vi "Get Type Code (Variant).vi"(6 "error in (no error)":errorcluster, 9 "value":variant) -> (0 "error out":errorcluster, 2 "type code":T1=enum."Bool", 3 "value dup":variant)   [LabVIEW 2020, in "Value.lvlib"]
uses:
  Value.lvlib
  Type Code.ctl
  <vilib>/Utility/Data Type/NI_Data Type.lvlib
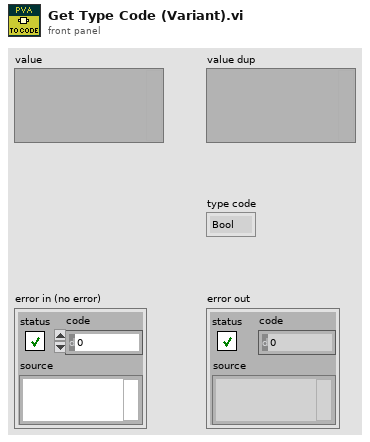
[diagram p1: front panel]
types:
  T1 = typedef "Value.lvlib/Type Code.ctl" = enum8{"Null", "Bool", "BoolA", "Int8", "Int8A", "Int16", "Int16A", "Int32", "Int32A", "Int64", "Int64A", "UInt8", "UInt8A", "UInt16", "UInt16A", "UInt32", "UInt32A", "UInt64", "UInt64A", "Float32", "Float32A", "Float64", "Float64A", "String", "StringA", "Struct", "StructA", "Union", "UnionA", "Any", "AnyA"}
  T2 = typedef "NI_Data Type.lvlib/Data Type.ctl" = enum8{"Invalid Type", "Void", "I8", "I16", "I32", "I64", "U8", "U16", "U32", "U64", "Single Float", "Double Float", "Extended Float", "Single Complex", "Double Complex", "Extended Complex", "Enum U8", "Enum U16", "Enum U32", "Enum U64", "Single Float With Unit", "Double Float With Unit", "Extended Float With Unit", "Single Complex with Unit", "Double Complex with Unit", "Extended Complex with Unit", "Boolean", "String", "Path", "Picture", "Tag", "Array", "Cluster", "Variant", "LV Variant", "Waveform", "Timestamp", "Digital Waveform", "Digital Data", "ExpressData", "Refnum", "External Data", "VI", "Poly VI", "LabVIEW Class Instance", "Fixed Point", "Set Collection", "Map Collection"}
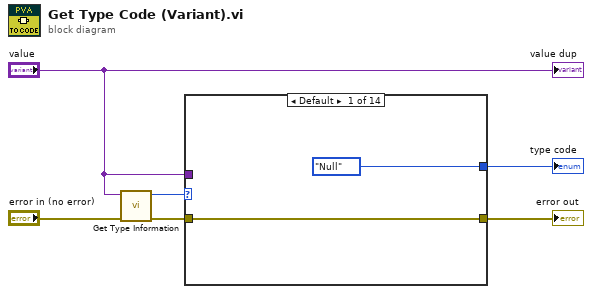
[diagram p0: block diagram]
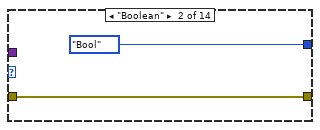
[diagram p2: hidden frame]
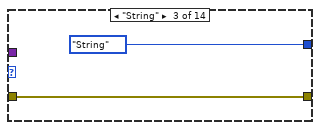
[diagram p3: hidden frame]
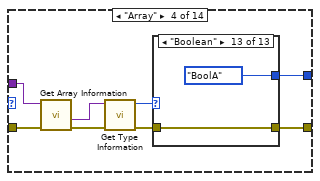
[diagram p4: hidden frame]
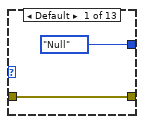
[diagram p5: hidden frame]
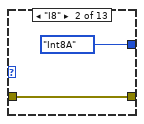
[diagram p6: hidden frame]
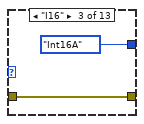
[diagram p7: hidden frame]
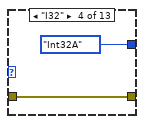
[diagram p8: hidden frame]
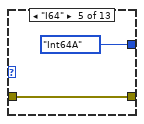
[diagram p9: hidden frame]
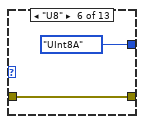
[diagram p10: hidden frame]
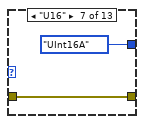
[diagram p11: hidden frame]
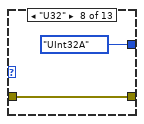
[diagram p12: hidden frame]
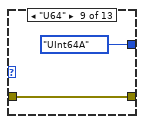
[diagram p13: hidden frame]
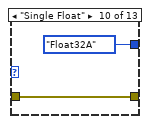
[diagram p14: hidden frame]
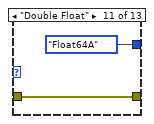
[diagram p15: hidden frame]
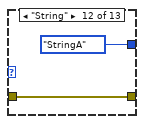
[diagram p16: hidden frame]
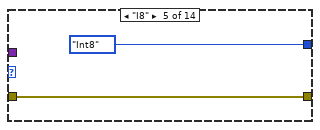
[diagram p17: hidden frame]
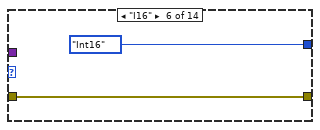
[diagram p18: hidden frame]
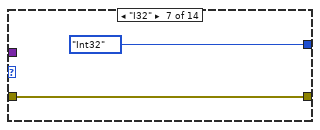
[diagram p19: hidden frame]
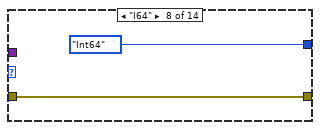
[diagram p20: hidden frame]
diagram:
  n1 = call <vilib>:"Get Type Information.vi"("error in (no error)"="error in (no error)", "variant"="value") -> ("error out"=w5:errorcluster, "type"=w2:T2)  [unwired: 5 in, 3 out]
  n2 = case shown="Default" w2 {
    tunnel: w5 -> [w7 w10 w12 w20 w48 w50 w52 w54 w56 w58 w60 w62 w64 w66]
    tunnel: [w7 w10 w12 w15 w48 w50 w52 w54 w56 w58 w60 w62 w64 w66] -> w4
    tunnel: [Type_Code."Null" ("Enum") Type_Code."Bool" ("Enum") Type_Code."String" ("Enum") w13 Type_Code."Int8" ("Enum") Type_Code."Int16" ("Enum") Type_Code."Int32" ("Enum") Type_Code."Int64" ("Enum") Type_Code."UInt8" ("Enum") Type_Code."UInt16" ("Enum") Type_Code."UInt32" ("Enum") Type_Code."UInt64" ("Enum") Type_Code."Float32" ("Enum") Type_Code."Float64" ("Enum")] -> w3
    tunnel: "value" -> [_ _ _ w19 _ _ _ _ _ _ _ _ _ _]
    frame Default {
    }
    frame "Boolean" {
    }
    frame "String" {
    }
    frame "Array" {
      n3 = call <vilib>:"Get Array Information.vi"("error in (no error)"=w20, "variant"=w19) -> ("error out"=w18:errorcluster, "array element data type"=w17:variant)  [unwired: 6 in, 2 out]
      n4 = call <vilib>:"Get Type Information.vi"("error in (no error)"=w18, "variant"=w17) -> ("error out"=w16:errorcluster, "type"=w14:T2)  [unwired: 5 in, 3 out]
      n5 = case shown="\"Boolean\"" w14 {
        tunnel: w16 -> [w22 w24 w26 w28 w30 w32 w34 w36 w38 w40 w42 w44 w46]
        tunnel: [w22 w24 w26 w28 w30 w32 w34 w36 w38 w40 w42 w44 w46] -> w15
        tunnel: [Type_Code."Null" ("Enum") Type_Code."Int8A" ("Enum") Type_Code."Int16A" ("Enum") Type_Code."Int32A" ("Enum") Type_Code."Int64A" ("Enum") Type_Code."UInt8A" ("Enum") Type_Code."UInt16A" ("Enum") Type_Code."UInt32A" ("Enum") Type_Code."UInt64A" ("Enum") Type_Code."Float32A" ("Enum") Type_Code."Float64A" ("Enum") Type_Code."StringA" ("Enum") Type_Code."BoolA" ("Enum")] -> w13
        frame Default {
        }
        frame "I8" {
        }
        frame "I16" {
        }
        frame "I32" {
        }
        frame "I64" {
        }
        frame "U8" {
        }
        frame "U16" {
        }
        frame "U32" {
        }
        frame "U64" {
        }
        frame "Single Float" {
        }
        frame "Double Float" {
        }
        frame "String" {
        }
        frame "Boolean" {
        }
      }
    }
    frame "I8" {
    }
    frame "I16" {
    }
    frame "I32" {
    }
    frame "I64" {
    }
    frame "U8" {
    }
    frame "U16" {
    }
    frame "U32" {
    }
    frame "U64" {
    }
    frame "Single Float" {
    }
    frame "Double Float" {
    }
  }
  "type code" <- w3
  "error out" <- w4
  "value dup" <- "value"
